vi "Get Connector Pane image.vi"(8 "error in":errorcluster, 11 "VI in":refnum<vi>) -> (0 "error out":errorcluster, 2 "Connector pane Image":picture, 3 "Vi out":refnum<vi>)   [LabVIEW 2020, in "DQMH_API.lvlib"]
uses:
  DQMH_API.lvlib
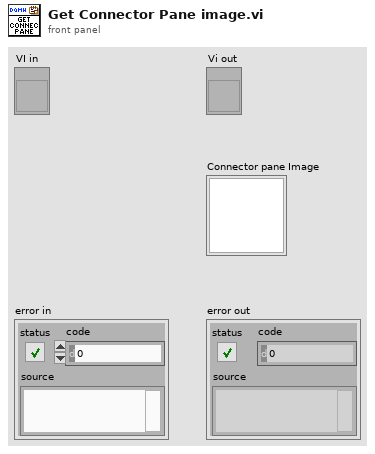
[diagram p1: front panel]
types:
  T1 = typedef "imagedata.ctl" = cluster{"image type":i32, "image depth":i32, "image":u8[], "mask":u8[], "colors":u32[], "Rectangle":cluster{"left":i16, "top":i16, "right":i16, "bottom":i16}}
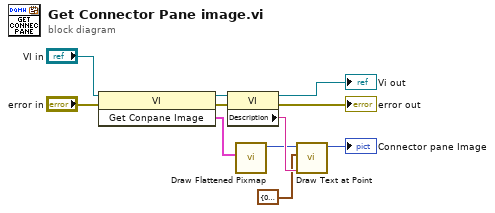
[diagram p0: block diagram]
diagram:
  n1 = invoke class="VI" method="Get Conpane Image"(reference="VI in", error in="error in") -> (reference out=w7:refnum<vi>, error out=w11:errorcluster, "Get Conpane Image"=w3:T1)  [unwired: 1 in]
  n2 = property class="VI"(reference=w7, error in=w11) -> (reference out=→"Vi out":refnum<vi>, error out=→"error out":errorcluster, "Description"=w8:string)
  n3 = call <vilib>:"Draw Flattened Pixmap.vi"("image data"=w3) -> ("new picture"=w4:picture)  [unwired: 8 in]
  n4 = call <vilib>:"Draw Text at Point.vi"("text"=w8, "origin"=cluster{"x":i16, "y":i16} {"x"=0, "y"=100}, "picture"=w4) -> ("new picture"=→"Connector pane Image":picture)  [unwired: 7 in, 1 out]
